vi "W&B Calculator (UPDATE)- Deniz Erselcan.vi"() -> ()   [LabVIEW 2026]
panel:
  out "System Message":string
  in  "Remaining Fuel":dbl
  in  "Start Button":bool
  out "Main Check":bool
  in  "Taxi Fuel":dbl
  in  "Stop":bool
  out "Landing Condition Arm Sum":dbl
  out "Landing Condition Mass Sum":dbl
  out "Landing Condition Moment Sum":dbl
  out "Landing Condition Indicator":bool
  out "Trip Fuel Arm Sum":dbl
  out "Trip Fuel Mass Sum":dbl
  out "Trip Fuel Moment Sum":dbl
  out "Trip Fuel Indicator":bool
  out "Take-Off Condition Arm Sum":dbl
  out "Take-Off Condition Mass Sum":dbl
  out "Take-Off Condition Moment Sum":dbl
  out "Take-Off Condition Indicator":bool
  out "Taxi Fuel Arm Sum":dbl
  out "Start/Taxi Fuel Mass Sum":dbl
  out "Taxi Fuel Moment Sum":dbl
  out "Taxi Indicator":bool
  out "Ramp Condition Arm Sum":dbl
  out "Ramp Condition Mass Sum":dbl
  out "Ramp Condition Moment Sum":dbl
  out "Ramp Condition Indicator":bool
  out "Fuel Loaded Arm Sum":dbl
  out "Fuel Loaded Mass Sum":dbl
  out "Fuel Loaded Moment Sum":dbl
  out "Fuel Loaded Indicator":bool
  out "Zero Fuel Arm Sum":dbl
  out "Zero Fuel Mass Sum":dbl
  out "Zero Fuel Moment Sum":dbl
  out "Zero Fuel Condition Indicator":bool
  out "Baggage Arm Sum":dbl
  out "Baggage Mass Sum":dbl
  out "Baggage Moment Sum":dbl
  out "Baggage Indicator":bool
  out "Rear Seat Arm Sum":dbl
  out "Rear Seat Mass Sum":dbl
  out "Rear Seat Moment Sum":dbl
  out "Rear Seat Indicator":bool
  out "Front Seat Arm Sum":dbl
  out "Front Seat Mass Sum":dbl
  out "Front Seat Moment Sum":dbl
  out "Front Seat Indicator":bool
  out "BEW Arm Sum":dbl
  out "BEW Mass Sum":dbl
  out "BEW Moment Sum":dbl
  out "BEW Indicator":bool
  out "Landing CG":dbl caption="CG"
  out "Take-Off CG":dbl caption="CG"
  out "Baggage Weight Check":dbl caption="kg"
  out "Landing Weight check":dbl caption="kg"
  out "Take-Off Weight Check":dbl caption="kg"
  out "Ramp Weight Check":dbl caption="kg"
  out "Landing CG Check":bool
  out "Take-Off CG Check":bool
  out "Baggage Check":bool
  out "Landing Weight Check":bool
  out "Take-Off Check":bool
  out "Ramp Weight Check":bool
  in  "Trip Fuel":dbl
  in  "Baggage":dbl
  in  "Passenger 2 (Right)":dbl
  in  "Passenger 1 (Left)":dbl
  in  "Co-Pilot Weight":dbl
  in  "Pilot Weight":dbl
  in  "BEW Arm":dbl
  in  "Basic Emty Weight":dbl
  out "Envelope Graph":cluster{dbl[], dbl[]}[](graph)
  # "Flight Crew"
  # "W & B Check"
  # "Aircraft Empty Weight"
  # "Pilot"
  # "Basic Empty Weight"
  # "kg"
  # "kg"
  # "kg"
  # "BEW Arm"
  # "Co-Pilot"
  # "in"
  # "Baggage"
  # "Passengers"
  # "App Control"
  # "Baggage"
  # "kg"
  # "Passenger 1 (Left)"
  # "kg"
  # "kg"
  # "Passenger 2 (Right)"
  # "System Message"
  # "CG Envelope Graph"
  # "Fuel (Avgas 100LL)"
  # "Loading Summary"
  # "Taxi Fuel"
  # "US Gal"
  # "MTOW"
  # "Trip Fuel"
  # "Basic Empty Weight"
  # "US Gal"
  # "Front Seat (Crew)"
  # "Reserve Fuel"
  # "US Gal"
  # "Rear Seat (Passengers)"
  # "Baggage"
  # "Limit Checks"
  # "Zero Fuel Condition"
  # "Ramp Weight"
  # "Fuel Loaded"
  # "Take-Off Weight"
  # "Ramp Condition"
  # "Landing Weight"
  # "Taxi Fuel"
  # "Baggage Weight"
  # "Take-Off Condition"
  # "Take-Off CG"
  # "Trip Fuel"
  # "Landing CG"
  # "Landing Condition"
  # "● Zero Fuel   ● Ramp   ● Take-Off   ● Landing"
  # "Item                                                     Mass(kg) Arm(in)  Moment   Status"
  # "Beechcraft Bonanza  — Weight & Balance Calculator"
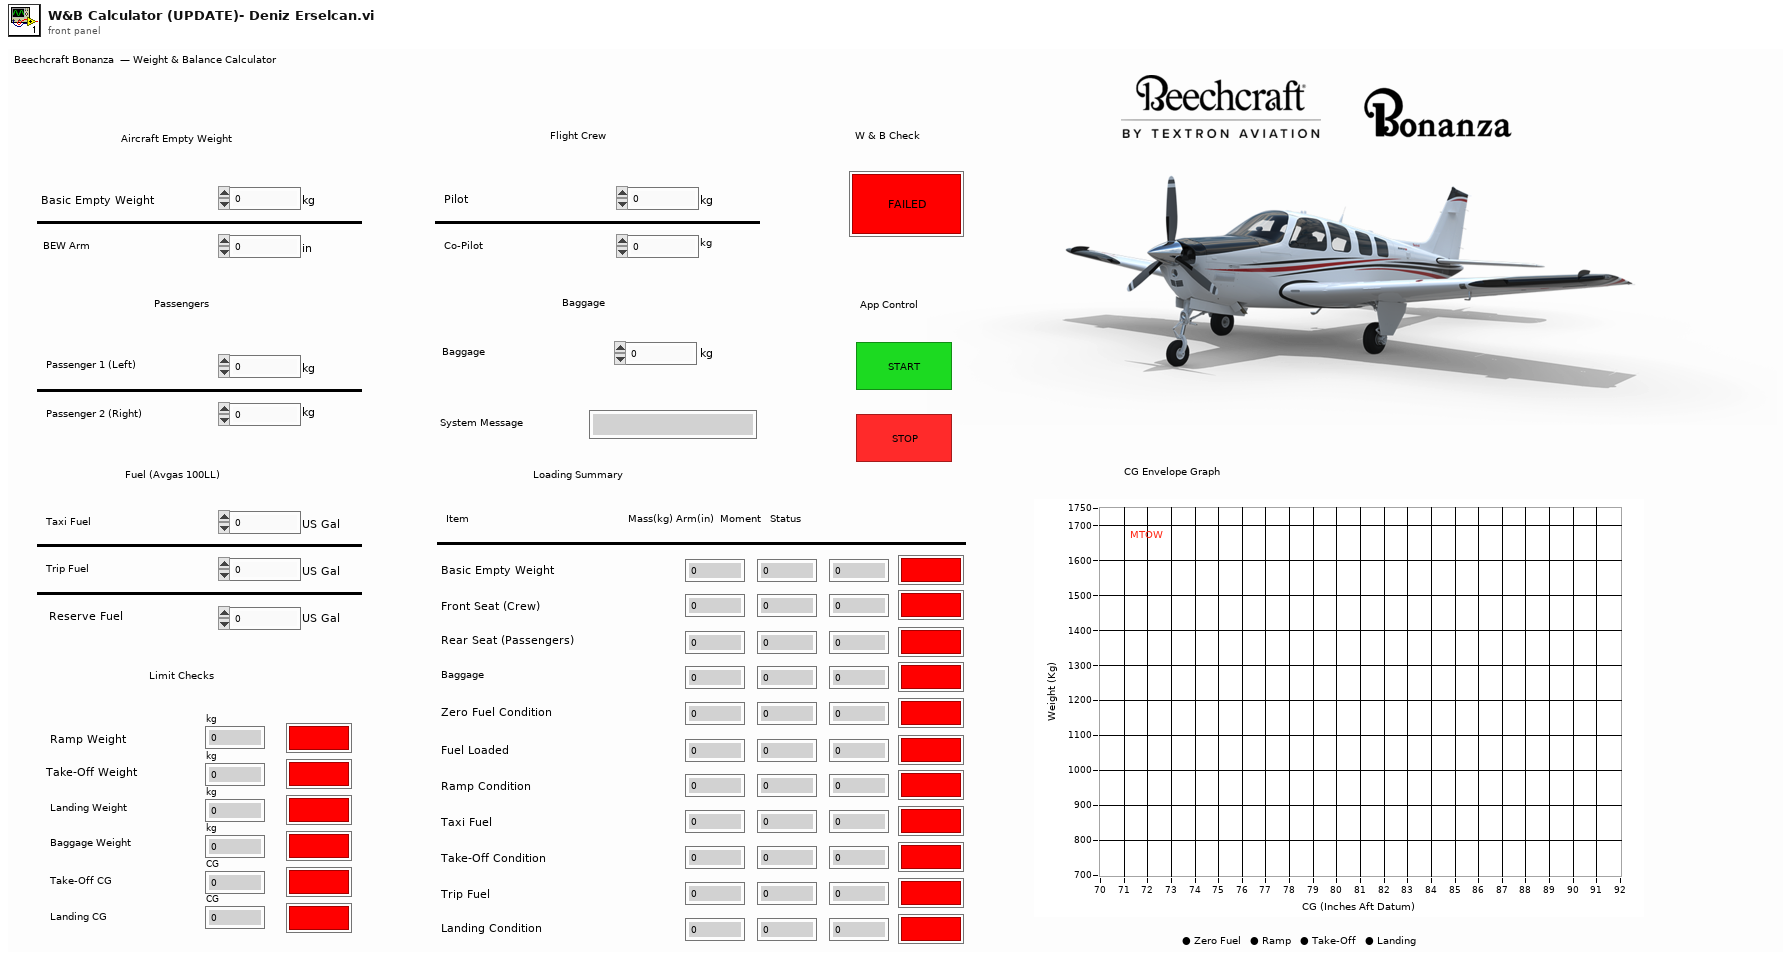
[diagram p1: front panel]
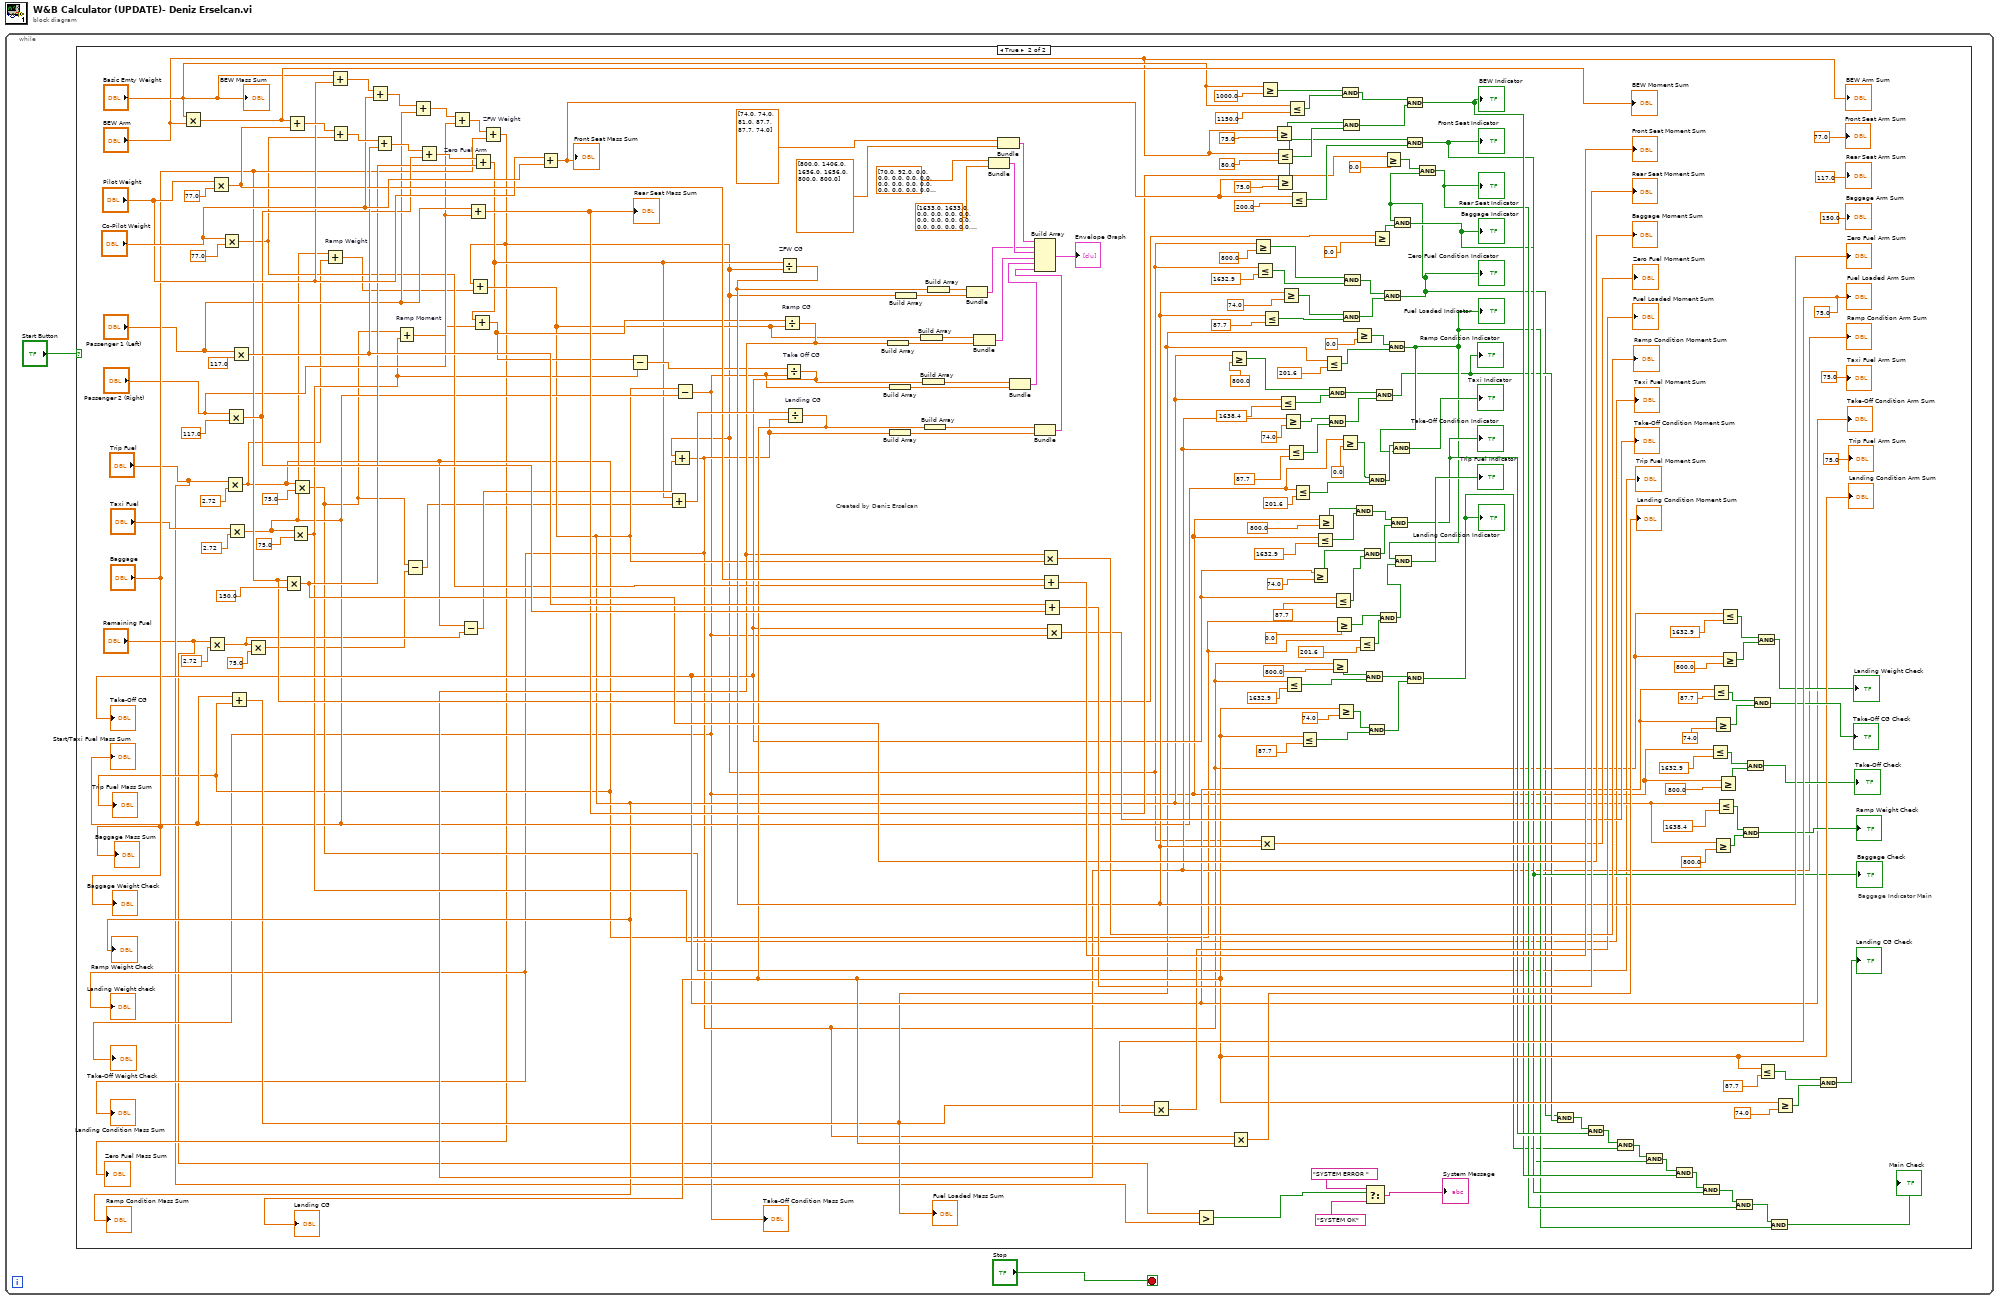
[diagram p0: block diagram]
diagram:
  n1 = while {
    stop <- "Stop" stop-if-true
    n2 = case shown="True" "Start Button" {
      frame False {
      }
      frame True {
        w153 = 75.0
        # "Baggage Indıcator Main"
        # "Created by Deniz Erselcan"
        n3 = Multiply(x="Basic Emty Weight", y="BEW Arm") -> (x*y=w165:dbl)
        "BEW Moment Sum" <- w165
        n4 = Multiply(x="Remaining Fuel", y=2.72) -> (x*y=w20:dbl)
        n5 = Multiply(x="Pilot Weight", y=77.0) -> (x*y=w164:dbl)
        n6 = Multiply(x="Co-Pilot Weight", y=77.0) -> (x*y=w32:dbl)
        n7 = Multiply(x="Trip Fuel", y=2.72) -> (x*y=w21:dbl)
        "Trip Fuel Mass Sum" <- w21
        n8 = Multiply(x="Passenger 2 (Right)", y=117.0) -> (x*y=w161:dbl)
        n9 = Multiply(x="Taxi Fuel", y=2.72) -> (x*y=w29:dbl)
        "Start/Taxi Fuel Mass Sum" <- w29
        n10 = Add(x=w29, y=w21) -> (x+y=w24:dbl)
        "Fuel Loaded Mass Sum" <- w24
        n11 = Multiply(x="Passenger 1 (Left)", y=117.0) -> (x*y=w162:dbl)
        n12 = Multiply(x=w20, y=75.0) -> (x*y=w18:dbl)
        n13 = Multiply(x="Baggage", y=150.0) -> (x*y=w159:dbl)
        "Baggage Moment Sum" <- w159
        n14 = Add(x=w165, y=w164) -> (x+y=w196:dbl)
        n15 = Multiply(x=w29, y=75.0) -> (x*y=w31:dbl)
        "Taxi Fuel Moment Sum" <- w31
        n16 = Multiply(x=w21, y=75.0) -> (x*y=w19:dbl)
        "Trip Fuel Moment Sum" <- w19
        n17 = Add "Ramp Weight"(x=w29, y=w21) -> (x+y=w25:dbl)
        n18 = Add(x="Basic Emty Weight", y="Pilot Weight") -> (x+y=w200:dbl)
        n19 = Add(x=w196, y=w32) -> (x+y=w195:dbl)
        n20 = Add(x=w200, y="Co-Pilot Weight") -> (x+y=w199:dbl)
        n21 = Add(x=w195, y=w162) -> (x+y=w194:dbl)
        n22 = Add "Ramp Moment"(x=w19, y=w31) -> (x+y=w27:dbl)
        n23 = Subtract(x=w19, y=w18) -> (x-y=w13:dbl)
        n24 = Add(x=w199, y="Passenger 1 (Left)") -> (x+y=w198:dbl)
        n25 = Add(x=w194, y=w161) -> (x+y=w193:dbl)
        n26 = Add(x=w198, y="Passenger 2 (Right)") -> (x+y=w197:dbl)
        n27 = Subtract(x=w21, y=w20) -> (x-y=w14:dbl)
        n28 = Add(x="Passenger 1 (Left)", y="Passenger 2 (Right)") -> (x+y=w133:dbl)
        "Rear Seat Mass Sum" <- w133
        n29 = Add "Zero Fuel Arm"(x=w193, y=w159) -> (x+y=w12:dbl)
        n30 = Add(x=w12, y=w27) -> (x+y=w28:dbl)
        n31 = Add "ZFW Weight"(x=w197, y="Baggage") -> (x+y=w11:dbl)
        "Zero Fuel Mass Sum" <- w11
        n32 = Add(x=w11, y=w25) -> (x+y=w26:dbl)
        "Ramp Weight Check" <- w26
        "Ramp Condition Mass Sum" <- w26
        n33 = Add(x="Pilot Weight", y="Co-Pilot Weight") -> (x+y=w136:dbl)
        "Front Seat Mass Sum" <- w136
        n34 = Subtract(x=w28, y=w31) -> (x-y=w15:dbl)
        n35 = Add(x=w12, y=w13) -> (x+y=w181:dbl)
        n36 = Add(x=w11, y=w14) -> (x+y=w17:dbl)
        "Landing Weight check" <- w17
        "Landing Condition Mass Sum" <- w17
        n37 = Subtract(x=w26, y=w29) -> (x-y=w16:dbl)
        "Take-Off Weight Check" <- w16
        "Take-Off Condition Mass Sum" <- w16
        n38 = Divide "ZFW CG"(x=w12, y=w11) -> (x/y=w119:dbl)
        "Zero Fuel Arm Sum" <- w119
        n39 = Divide "Ramp CG"(x=w28, y=w26) -> (x/y=w30:dbl)
        "Ramp Condition Arm Sum" <- w30
        n40 = Divide "Take Off CG"(x=w15, y=w16) -> (x/y=w51:dbl)
        "Take-Off CG" <- w51
        "Take-Off Condition Arm Sum" <- w51
        n41 = Divide "Landing CG"(x=w181, y=w17) -> (x/y=w68:dbl)
        "Landing CG" <- w68
        "Landing Condition Arm Sum" <- w68
        n42 = Build Array(w30) -> (w189:dbl[])
        n43 = Build Array(w16) -> (w182:dbl[])
        n44 = Build Array(w17) -> (w179:dbl[])
        n45 = Build Array(w11) -> (w191:dbl[])
        n46 = Build Array(w26) -> (w188:dbl[])
        n47 = Build Array(w51) -> (w183:dbl[])
        n48 = Build Array(w68) -> (w180:dbl[])
        n49 = Build Array(w119) -> (w192:dbl[])
        n50 = Bundle(w192, w191) -> (w190:cluster{dbl[], dbl[]})  [unwired: 1 in]
        n51 = Bundle(w189, w188) -> (w187:cluster{dbl[], dbl[]})  [unwired: 1 in]
        n52 = Bundle(dbl[] [70.0, 92.0, 0.0, 0.0, 0.0, 0.0, 0.0, 0.0, 0.0, 0.0, 0.0, 0.0, 0.0, 0.0, 0.0, 0.0, 0.0, 0.0, 0.0, 0.0, 0.0, 0.0, 0.0, 0.0, 0.0, 0.0, 0.0, 0.0, 0.0, 0.0, 0.0, 0.0, 0.0, 0.0, 0.0, 0.0, 0.0, 0.0, 0.0, 0.0, 0.0, 0.0, 0.0, 0.0, 0.0, 0.0, 0.0, 0.0, 0.0, 0.0, 0.0, 0.0, 0.0, 0.0, 0.0, 0.0, 0.0, 0.0, 0.0, 0.0, 0.0, 0.0, 0.0, 0.0, 0.0, 0.0, 0.0, 0.0, 0.0, 0.0, 0.0, 0.0, 0.0, 0.0, 0.0, 0.0, 0.0, 77.0], dbl[] [1633.0, 1633.0, 0.0, 0.0, 0.0, 0.0, 0.0, 0.0, 0.0, 0.0, 0.0, 0.0, 0.0, 0.0, 0.0, 0.0, 0.0, 0.0, 0.0, 0.0, 0.0, 0.0, 0.0, 0.0, 0.0, 0.0, 0.0, 0.0, 0.0, 0.0, 0.0, 0.0, 0.0, 0.0, 0.0, 0.0, 0.0, 0.0, 0.0, 0.0, 0.0, 0.0, 0.0, 0.0, 0.0, 0.0, 0.0, 0.0, 0.0, 0.0, 0.0, 0.0, 0.0, 0.0, 0.0, 0.0, 0.0, 0.0, 0.0, 0.0, 0.0, 0.0, 0.0, 0.0, 0.0, 0.0, 0.0, 0.0, 0.0, 0.0, 0.0, 0.0, 0.0, 0.0, 0.0, 0.0, 0.0, 0.0, 0.0, 0.0, 0.0, 0.0, 0.0, 0.0, 0.0, 0.0, 0.0, 0.0, 0.0, 0.0, 0.0, 0.0, 0.0, 0.0, 0.0, 0.0, 0.0, 0.0, 0.0, 0.0, 0.0, 0.0, 0.0, 0.0, 0.0, 0.0, 0.0, 0.0, 0.0, 0.0, 0.0, 0.0, 0.0, 0.0, 0.0, 0.0, 0.0, 0.0, 0.0, 0.0, 0.0, 0.0, 0.0, 0.0, 0.0, 0.0, 0.0, 0.0, 0.0, 0.0, 0.0, 0.0, 0.0, 0.0, 0.0, 0.0, 0.0, 0.0, 0.0, 0.0, 0.0, 0.0, 0.0, 0.0, 0.0, 0.0, 0.0, 0.0, 0.0, 0.0, 0.0, 0.0, 0.0, 0.0, 0.0, 0.0, 0.0, 0.0, 0.0, 0.0, 0.0, 0.0, 0.0, 0.0, 0.0, 0.0, 0.0, 0.0, 0.0, 0.0, 0.0, 0.0, 0.0, 0.0, 0.0, 0.0, 0.0, 0.0, 0.0, 0.0, 0.0, 0.0, 0.0, 0.0, 0.0, 0.0, 0.0, 0.0, 0.0, 0.0, 0.0, 0.0, 0.0, 0.0, 0.0, 0.0, 0.0, 0.0, 0.0, 0.0, 0.0, 0.0, 0.0, 0.0, 0.0, 0.0, 0.0, 0.0, 0.0, 0.0, 0.0, 0.0, 0.0, 0.0, 0.0, 0.0, 0.0, 0.0, 0.0, 0.0, 0.0, 0.0, 0.0, 0.0, 0.0, 0.0, 0.0, 0.0, 0.0, 0.0, 0.0, 0.0, 0.0, 0.0, 0.0, 0.0, 0.0, 0.0, 0.0, 0.0, 0.0, 0.0, 0.0, 0.0, 0.0, 0.0, 0.0, 0.0, 0.0, 0.0, 0.0, 0.0, 0.0, 0.0, 0.0, 0.0, 0.0, 0.0, 0.0, 0.0, 0.0, 0.0, 0.0, 0.0, 0.0, 0.0, 0.0, 0.0, 0.0, 0.0, 0.0, 0.0, 0.0, 0.0, 0.0, 0.0, 0.0, 0.0, 0.0, 0.0, 0.0, 0.0, 0.0, 0.0, 0.0, 0.0, 0.0, 0.0, 0.0, 0.0, 0.0, 0.0, 0.0, 0.0, 0.0, 0.0, 0.0, 0.0, 0.0, 0.0, 0.0, 0.0, 0.0, 0.0, 0.0, 0.0, 0.0, 0.0, 0.0, 0.0, 0.0, 0.0, 0.0, 0.0, 0.0, 0.0, 0.0, 0.0, 0.0, 0.0, 0.0, 0.0, 0.0, 0.0, 0.0, 0.0, 0.0, 0.0, 0.0, 0.0, 0.0, 0.0, 0.0, 0.0, 0.0, 0.0, 0.0, 0.0, 0.0, 0.0, 0.0, 0.0, 0.0, 0.0, 0.0, 0.0, 0.0, 0.0, 0.0, 0.0, 0.0, 0.0, 0.0, 0.0, 0.0, 0.0, 0.0, 0.0, 0.0, 0.0, 0.0, 0.0, 0.0, 0.0, 0.0, 0.0, 0.0, 0.0, 0.0, 0.0, 0.0, 0.0, 0.0, 0.0, 0.0, 0.0, 0.0, 0.0, 0.0, 0.0, 0.0, 0.0, 0.0, 0.0, 0.0, 0.0, 0.0, 0.0, 0.0, 0.0, 0.0, 0.0, 0.0, 0.0, 0.0, 0.0, 0.0, 0.0, 0.0, 0.0, 0.0, 0.0, 0.0, 0.0, 0.0, 0.0, 0.0, 0.0, 0.0, 0.0, 0.0, 0.0, 0.0, 0.0, 0.0, 0.0, 0.0, 0.0, 0.0, 0.0, 0.0, 0.0, 0.0, 0.0, 0.0, 0.0, 0.0, 0.0, 0.0, 0.0, 0.0, 0.0, 0.0, 0.0, 0.0, 0.0, 0.0, 0.0, 0.0, 0.0, 0.0, 0.0, 0.0, 0.0, 0.0, 0.0, 0.0, 0.0, 0.0, 0.0, 0.0, 0.0, 0.0, 0.0, 0.0, 0.0, 0.0, 0.0, 0.0, 0.0, 0.0, 0.0, 0.0, 0.0, 0.0, 0.0, 0.0, 0.0, 0.0, 0.0, 0.0, 0.0, 0.0, 0.0, 0.0, 0.0, 0.0, 0.0, 0.0, 0.0, 0.0, 0.0, 0.0, 0.0, 0.0, 0.0, 0.0, 0.0, 0.0, 0.0, 0.0, 0.0, 0.0, 0.0, 0.0, 0.0, 0.0, 0.0, 0.0, 0.0, 0.0, 0.0, 0.0, 0.0, 0.0, 0.0, 0.0, 0.0, 0.0, 0.0, 0.0, 0.0, 0.0, 0.0, 0.0, 0.0, 0.0, 0.0, 0.0, 0.0, 0.0, 0.0, 0.0, 0.0, 0.0, 0.0, 0.0, 0.0, 0.0, 0.0, 0.0, 0.0, 0.0, 0.0, 0.0, 0.0, 0.0, 0.0, 0.0, 0.0, 0.0, 0.0, 0.0, 0.0, 0.0, 0.0, 0.0, 0.0, 0.0, 0.0, 0.0, 0.0, 0.0, 0.0, 0.0, 0.0, 0.0, 0.0, 0.0, 0.0, 0.0, 0.0, 0.0, 0.0, 0.0, 0.0, 0.0, 0.0, 0.0, 0.0, 0.0, 0.0, 0.0, 0.0, 0.0, 0.0, 0.0, 0.0, 0.0, 0.0, 0.0, 0.0, 0.0, 0.0, 0.0, 0.0, 0.0, 0.0, 0.0, 0.0, 0.0, 0.0, 0.0, 0.0, 0.0, 0.0, 0.0, 0.0, 0.0, 0.0, 0.0, 0.0, 0.0, 0.0, 0.0, 0.0, 0.0, 0.0, 0.0, 0.0, 0.0, 0.0, 0.0, 0.0, 0.0, 0.0, 0.0, 0.0, 0.0, 0.0, 0.0, 0.0, 0.0, 0.0, 0.0, 0.0, 0.0, 0.0, 0.0, 0.0, 0.0, 0.0, 0.0, 0.0, 0.0, 0.0, 0.0, 0.0, 0.0, 0.0, 0.0, 0.0, 0.0, 0.0, 0.0, 0.0, 0.0, 0.0, 0.0, 0.0, 0.0, 0.0, 0.0, 0.0, 0.0, 0.0, 0.0, 0.0, 0.0, 0.0, 0.0, 0.0, 0.0, 0.0, 0.0, 0.0, 0.0, 0.0, 0.0, 0.0, 0.0, 0.0, 0.0, 0.0, 0.0, 0.0, 0.0, 0.0, 0.0, 0.0, 0.0, 0.0, 0.0, 0.0, 0.0, 0.0, 0.0, 0.0, 0.0, 0.0, 0.0, 0.0, 0.0, 0.0, 0.0, 0.0, 0.0, 0.0, 0.0, 0.0, 0.0, 0.0, 0.0, 0.0, 0.0, 0.0, 0.0, 0.0, 0.0, 0.0, 0.0, 0.0, 0.0, 0.0, 0.0, 0.0, 0.0, 0.0, 0.0, 0.0, 0.0, 0.0, 0.0, 0.0, 0.0, 0.0, 0.0, 0.0, 0.0, 0.0, 0.0, 0.0, 0.0, 0.0, 0.0, 0.0, 0.0, 0.0, 0.0, 0.0, 0.0, 0.0, 0.0, 0.0, 0.0, 0.0, 0.0, 0.0, 0.0, 0.0, 0.0, 0.0, 0.0, 0.0, 0.0, 0.0, 0.0, 0.0, 0.0, 0.0, 0.0, 0.0, 0.0, 0.0, 0.0, 0.0, 0.0, 0.0, 0.0, 0.0, 0.0, 0.0, 0.0, 0.0, 0.0, 0.0, 0.0, 0.0, 0.0, 0.0, 0.0, 0.0, 0.0, 0.0, 0.0, 0.0, 0.0, 0.0, 0.0, 0.0, 0.0, 0.0, 0.0, 0.0, 0.0, 0.0, 0.0, 0.0, 0.0, 0.0, 0.0, 0.0, 0.0, 0.0, 0.0, 0.0, 0.0, 0.0, 0.0, 0.0, 0.0, 0.0, 0.0, 0.0, 0.0, 0.0, 0.0, 0.0, 0.0, 0.0, 0.0, 0.0, 0.0, 0.0, 0.0, 0.0, 0.0, 0.0, 0.0, 0.0, 0.0, 0.0, 0.0, 0.0, 0.0, 0.0, 0.0, 0.0, 0.0, 0.0, 0.0, 0.0, 0.0, 0.0, 0.0, 0.0, 0.0, 0.0, 0.0, 0.0, 0.0, 0.0, 0.0, 0.0, 0.0, 0.0, 0.0, 0.0, 0.0, 0.0, 0.0, 0.0, 0.0, 0.0, 0.0, 0.0, 0.0, 0.0, 0.0, 0.0, 0.0, 0.0, 0.0, 0.0, 0.0, 0.0, 0.0, 0.0, 0.0, 0.0, 0.0, 0.0, 0.0, 0.0, 0.0, 0.0, 0.0, 0.0, 0.0, 0.0, 0.0, 0.0, 0.0, 0.0, 0.0, 0.0, 0.0, 0.0, 0.0, 0.0, 0.0, 0.0, 0.0, 0.0, 0.0, 0.0, 0.0, 0.0, 0.0, 0.0, 0.0, 0.0, 0.0, 0.0, 0.0, 0.0, 0.0, 0.0, 0.0, 0.0, 0.0, 0.0, 0.0, 0.0, 0.0, 0.0, 0.0, 0.0, 0.0, 0.0, 0.0, 0.0, 0.0, 0.0, 0.0, 0.0, 0.0, 0.0, 0.0, 0.0, 0.0, 0.0, 0.0, 0.0, 0.0, 0.0, 0.0, 0.0, 0.0, 0.0, 0.0, 0.0, 0.0, 0.0, 0.0, 0.0, 0.0, 0.0, 0.0, 0.0, 0.0, 0.0, 0.0, 0.0, 0.0, 0.0, 0.0, 0.0, 0.0, 0.0, 0.0, 0.0, 0.0, 0.0, 0.0, 0.0, 0.0, 0.0, 0.0, 0.0, 0.0, 0.0, 0.0, 0.0, 0.0, 0.0, 0.0, 0.0, 0.0, 0.0, 0.0, 0.0, 0.0, 0.0, 0.0, 0.0, 0.0, 0.0, 0.0, 0.0, 0.0, 0.0, 0.0, 0.0, 0.0, 0.0, 0.0, 0.0, 0.0, 0.0, 0.0, 0.0, 0.0, 0.0, 0.0, 0.0, 0.0, 0.0, 0.0, 0.0, 0.0, 0.0, 0.0, 0.0, 0.0, 0.0, 0.0, 0.0, 0.0, 0.0, 0.0, 0.0, 0.0, 0.0, 0.0, 0.0, 0.0, 0.0, 0.0, 0.0, 0.0, 0.0, 0.0, 0.0, 0.0, 0.0, 0.0, 0.0, 0.0, 0.0, 0.0, 0.0, 0.0, 0.0, 0.0, 0.0, 0.0, 0.0, 0.0, 0.0, 0.0, 0.0, 0.0, 0.0, 0.0, 0.0, 0.0, 0.0, 0.0, 0.0, 0.0, 0.0, 0.0, 0.0, 0.0, 0.0, 0.0, 0.0, 0.0, 0.0, 0.0, 0.0, 0.0, 0.0, 0.0, 0.0, 0.0, 0.0, 0.0, 0.0, 0.0, 0.0, 0.0, 0.0, 0.0, 0.0, 0.0, 0.0, 0.0, 0.0, 0.0, 0.0, 0.0, 0.0, 0.0, 0.0, 0.0, 0.0, 0.0, 0.0, 0.0, 0.0, 0.0, 0.0, 0.0, 0.0, 0.0, 0.0, 0.0, 0.0, 0.0, 0.0, 0.0, 0.0, 0.0, 0.0, 0.0, 0.0, 0.0, 0.0, 0.0, 0.0, 0.0, 0.0, 0.0, 0.0, 0.0, 0.0, 0.0, 0.0, 0.0, 0.0, 0.0, 0.0, 0.0, 0.0, 0.0, 0.0, 0.0, 0.0, 0.0, 0.0, 0.0, 0.0, 0.0, 0.0, 0.0, 0.0, 0.0, 0.0, 0.0, 0.0, 0.0, 0.0, 0.0, 0.0, 0.0, 0.0, 0.0, 0.0, 0.0, 0.0, 0.0, 0.0, 0.0, 0.0, 0.0, 0.0, 0.0, 0.0, 0.0, 0.0, 0.0, 0.0, 0.0, 0.0, 0.0, 0.0, 0.0, 0.0, 0.0, 0.0, 0.0, 0.0, 0.0, 0.0, 0.0, 0.0, 0.0, 0.0, 0.0, 0.0, 0.0, 0.0, 0.0, 0.0, 0.0, 0.0, 0.0, 0.0, 0.0, 0.0, 0.0, 0.0, 0.0, 0.0, 0.0, 0.0, 0.0, 0.0, 0.0, 0.0, 0.0, 0.0, 0.0, 0.0, 0.0, 0.0, 0.0, 0.0, 0.0, 0.0, 0.0, 0.0, 0.0, 0.0, 0.0, 0.0, 0.0, 0.0, 0.0, 0.0, 0.0, 0.0, 0.0, 0.0, 0.0, 0.0, 0.0, 0.0, 0.0, 0.0, 0.0, 0.0, 0.0, 0.0, 0.0, 0.0, 0.0, 0.0, 0.0, 0.0, 0.0, 0.0, 0.0, 0.0, 0.0, 0.0, 0.0, 0.0, 0.0, 0.0, 0.0, 0.0, 0.0, 0.0, 0.0, 0.0, 0.0, 0.0, 0.0, 0.0, 0.0, 0.0, 0.0, 0.0, 0.0, 0.0, 0.0, 0.0, 0.0, 0.0, 0.0, 0.0, 0.0, 0.0, 0.0, 0.0, 0.0, 0.0, 0.0, 0.0, 0.0, 0.0, 0.0, 0.0, 0.0, 0.0, 0.0, 0.0, 0.0, 0.0, 0.0, 0.0, 0.0, 0.0, 0.0, 0.0, 0.0, 0.0, 1320.0]) -> (w209:cluster{dbl[], dbl[]})  [unwired: 1 in]
        n53 = Bundle(dbl[] [74.0, 74.0, 81.0, 87.7, 87.7, 74.0], dbl[] [800.0, 1406.0, 1656.0, 1656.0, 800.0, 800.0]) -> (w212:cluster{dbl[], dbl[]})  [unwired: 1 in]
        n54 = Bundle(w183, w182) -> (w184:cluster{dbl[], dbl[]})  [unwired: 1 in]
        n55 = Bundle(w180, w179) -> (w178:cluster{dbl[], dbl[]})  [unwired: 1 in]
        n56 = Build Array(w212, w190, w209, w187, w184, w178) -> (→"Envelope Graph":cluster{dbl[], dbl[]}[])
        n57 = Multiply(x=w30, y=w26) -> (x*y=→"Ramp Condition Moment Sum":dbl)
        n58 = Add(x=w164, y=w32) -> (x+y=→"Front Seat Moment Sum":dbl)
        n59 = Add(x=w162, y=w161) -> (x+y=→"Rear Seat Moment Sum":dbl)
        n60 = Multiply(x=w51, y=w16) -> (x*y=→"Take-Off Condition Moment Sum":dbl)
        n61 = Multiply(x=w24, y=w153) -> (x*y=→"Fuel Loaded Moment Sum":dbl)
        n62 = Greater?(x="Remaining Fuel", y="Trip Fuel") -> (0:w3:bool)
        n63 = Greater Or Equal?(x=w26, y=800.0) -> (x >= y?=w114:bool)
        n64 = Multiply(x=w17, y=w68) -> (x*y=→"Landing Condition Moment Sum":dbl)
        n65 = Greater Or Equal?(x=w11, y=800.0) -> (x >= y?=w129:bool)
        n66 = Less Or Equal?(x=w11, y=1632.9) -> (x <= y?=w128:bool)
        n67 = Multiply(x=w11, y=w119) -> (x*y=→"Zero Fuel Moment Sum":dbl)
        n68 = Greater Or Equal?(x="Basic Emty Weight", y=1000.0) -> (x >= y?=w150:bool)
        n69 = Less Or Equal?(x=w119, y=87.7) -> (x <= y?=w124:bool)
        n70 = Greater Or Equal?(x="BEW Arm", y=75.0) -> (x >= y?=w145:bool)
        n71 = Less Or Equal?(x="BEW Arm", y=80.0) -> (x <= y?=w141:bool)
        n72 = Greater Or Equal?(x=w136, y=75.0) -> (x >= y?=w140:bool)
        n73 = Less Or Equal?(x=w26, y=1638.4) -> (x <= y?=w113:bool)
        n74 = Greater Or Equal?(x=w119, y=74.0) -> (x >= y?=w125:bool)
        n75 = Greater Or Equal?(x=w30, y=74.0) -> (x >= y?=w110:bool)
        n76 = Less Or Equal?(x=w17, y=1632.9) -> (x <= y?=w85:bool)
        n77 = Less Or Equal?(x=w30, y=87.7) -> (x <= y?=w109:bool)
        n78 = Less Or Equal?(x="Basic Emty Weight", y=1150.0) -> (x <= y?=w149:bool)
        n79 = Less Or Equal?(x=w136, y=200.0) -> (x <= y?=w139:bool)
        n80 = Less Or Equal?(x=w29, y=201.6) -> (x <= y?=w103:bool)
        n81 = Less Or Equal?(x=w68, y=87.7) -> (x <= y?=w81:bool)
        n82 = Greater Or Equal?(x=w51, y=74.0) -> (x >= y?=w96:bool)
        n83 = Less Or Equal?(x=w16, y=1632.9) -> (x <= y?=w99:bool)
        n84 = Greater Or Equal?(x=w16, y=800.0) -> (x >= y?=w100:bool)
        n85 = Less Or Equal?(x=w24, y=201.6) -> (x <= y?=w117:bool)
        n86 = And(x=w110, y=w109) -> (x .and. y?=w105:bool)
        n87 = And(x=w114, y=w113) -> (x .and. y?=w106:bool)
        n88 = Greater Or Equal?(x=w17, y=800.0) -> (x >= y?=w86:bool)
        n89 = Less Or Equal?(x=w51, y=87.7) -> (x <= y?=w95:bool)
        n90 = Greater Or Equal?(x=w21, y=0.0) -> (x >= y?=w90:bool)
        n91 = Greater Or Equal?(x=w68, y=74.0) -> (x >= y?=w82:bool)
        n92 = And(x=w150, y=w149) -> (x .and. y?=w144:bool)
        n93 = Greater Or Equal?(x=w29, y=0.0) -> (x >= y?=w104:bool)
        n94 = And(x=w145, y=w141) -> (x .and. y?=w143:bool)
        n95 = And(x=w125, y=w124) -> (x .and. y?=w120:bool)
        n96 = And(x=w129, y=w128) -> (x .and. y?=w121:bool)
        n97 = Greater Or Equal?(x=w24, y=0.0) -> (x >= y?=w118:bool)
        n98 = And(x=w100, y=w99) -> (x .and. y?=w92:bool)
        n99 = Less Or Equal?(x=w21, y=201.6) -> (x <= y?=w89:bool)
        n100 = And(x=w96, y=w95) -> (x .and. y?=w91:bool)
        n101 = And(x=w86, y=w85) -> (x .and. y?=w78:bool)
        n102 = Select(t="SYSTEM ERROR ", s=w3, f="SYSTEM OK") -> (s? t:f=→"System Message":string)
        n103 = And(x=w82, y=w81) -> (x .and. y?=w77:bool)
        n104 = And(x=w104, y=w103) -> (x .and. y?=w75:bool)
        n105 = Greater Or Equal?(x="Baggage", y=0.0) -> (x >= y?=w132:bool)
        n106 = And(x=w106, y=w105) -> (x .and. y?=w35:bool)
        "Ramp Condition Indicator" <- w35
        n107 = And(x=w90, y=w89) -> (x .and. y?=w76:bool)
        n108 = And(x=w121, y=w120) -> (x .and. y?=w10:bool)
        "Zero Fuel Condition Indicator" <- w10
        n109 = Greater Or Equal?(x=w133, y=0.0) -> (x >= y?=w135:bool)
        n110 = And(x=w118, y=w117) -> (x .and. y?=w39:bool)
        "Fuel Loaded Indicator" <- w39
        n111 = And(x=w92, y=w91) -> (x .and. y?=w48:bool)
        "Take-Off Condition Indicator" <- w48
        n112 = And(x=w75, y=w39) -> (x .and. y?=→"Taxi Indicator":bool)
        n113 = And(x=w10, y=w132) -> (x .and. y?=w36:bool)
        "Baggage Check" <- w36
        "Baggage Indicator" <- w36
        n114 = And(x=w39, y=w76) -> (x .and. y?=→"Trip Fuel Indicator":bool)
        n115 = And(x=w144, y=w143) -> (x .and. y?=w45:bool)
        "BEW Indicator" <- w45
        n116 = And(x=w140, y=w139) -> (x .and. y?=w43:bool)
        "Front Seat Indicator" <- w43
        n117 = And(x=w78, y=w77) -> (x .and. y?=w34:bool)
        "Landing Condition Indicator" <- w34
        n118 = And(x=w135, y=w10) -> (x .and. y?=w41:bool)
        "Rear Seat Indicator" <- w41
        n119 = And(x=w10, y=w35) -> (x .and. y?=w50:bool)
        n120 = And(x=w50, y=w48) -> (x .and. y?=w49:bool)
        n121 = And(x=w49, y=w34) -> (x .and. y?=w47:bool)
        n122 = And(x=w47, y=w36) -> (x .and. y?=w46:bool)
        n123 = And(x=w46, y=w45) -> (x .and. y?=w44:bool)
        n124 = And(x=w44, y=w43) -> (x .and. y?=w42:bool)
        n125 = Less Or Equal?(x=w16, y=1632.9) -> (x <= y?=w54:bool)
        n126 = Less Or Equal?(x=w51, y=87.7) -> (x <= y?=w72:bool)
        n127 = Greater Or Equal?(x=w51, y=74.0) -> (x >= y?=w71:bool)
        n128 = Greater Or Equal?(x=w26, y=800.0) -> (x >= y?=w59:bool)
        n129 = Less Or Equal?(x=w26, y=1638.4) -> (x <= y?=w58:bool)
        n130 = Greater Or Equal?(x=w16, y=800.0) -> (x >= y?=w55:bool)
        n131 = Greater Or Equal?(x=w17, y=800.0) -> (x >= y?=w63:bool)
        n132 = Less Or Equal?(x=w17, y=1632.9) -> (x <= y?=w62:bool)
        n133 = And(x=w42, y=w41) -> (x .and. y?=w40:bool)
        n134 = And(x=w58, y=w59) -> (x .and. y?=→"Ramp Weight Check":bool)
        n135 = And(x=w54, y=w55) -> (x .and. y?=→"Take-Off Check":bool)
        n136 = And(x=w72, y=w71) -> (x .and. y?=→"Take-Off CG Check":bool)
        n137 = And(x=w62, y=w63) -> (x .and. y?=→"Landing Weight Check":bool)
        n138 = Less Or Equal?(x=w68, y=87.7) -> (x <= y?=w67:bool)
        n139 = And(x=w40, y=w39) -> (x .and. y?=→"Main Check":bool)
        n140 = Greater Or Equal?(x=w68, y=74.0) -> (x >= y?=w66:bool)
        n141 = And(x=w67, y=w66) -> (x .and. y?=→"Landing CG Check":bool)
        "Baggage Weight Check" <- "Baggage"
        "BEW Mass Sum" <- "Basic Emty Weight"
        "BEW Arm Sum" <- "BEW Arm"
        "Front Seat Arm Sum" <- 77.0
        "Rear Seat Arm Sum" <- 117.0
        "Baggage Mass Sum" <- "Baggage"
        "Baggage Arm Sum" <- 150.0
        "Fuel Loaded Arm Sum" <- w153
        "Taxi Fuel Arm Sum" <- 75.0
        "Trip Fuel Arm Sum" <- 75.0
      }
    }
  }
